vi "Create List Of FPGA in this Schedule.vi"(8 "error in (no error)":errorcluster, 11 "Schedule in":refnum<class "Schedule.lvclass">) -> (0 "error out":errorcluster, 3 "Schedule out":refnum<class "Schedule.lvclass">)   [LabVIEW 2020, in "TALOS.lvlib" / "Run Utilities.lvlib" / "Schedule.lvclass"]
doc: "Go over the entire schedule and create a list of Kaslis that are used in the Schedule"
uses:
  Schedule.lvclass
  Schedule.lvclass/Schedule.ctl
  Get List Of Kaslis in this Schedule.vi/21cbf78c-3c17-4340-8c34-790405437e2d.vi/d4db2432-cc9c-482c-8957-dac855435ef6.vi
  Get List Of Kaslis in this Schedule.vi/21cbf78c-3c17-4340-8c34-790405437e2d.vi/86fbf154-bd7b-49a2-8ab2-a837b2a95f24.vi
  Get List Of Kaslis in this Schedule.vi/21cbf78c-3c17-4340-8c34-790405437e2d.vi/3b95b01e-1ec2-4565-bcd9-7606a5281010.vi
  Get List Of Kaslis in this Schedule.vi/21cbf78c-3c17-4340-8c34-790405437e2d.vi/96a08935-737a-44b2-979c-a81d56408f7e.vi
  Get List Of Kaslis in this Schedule.vi/fc6b4163-bfed-4ba7-be7f-d257c96f9c4b.vi/c0db33a9-eb6c-44d9-b982-8563e05d2734.vi
  Get List Of Kaslis in this Schedule.vi/fc6b4163-bfed-4ba7-be7f-d257c96f9c4b.vi/ae3535a8-0066-4e8d-a5de-b07ac05a7c65.vi
  Get List Of Kaslis in this Schedule.vi/fc6b4163-bfed-4ba7-be7f-d257c96f9c4b.vi/dda8e586-731b-4197-ad83-6a4d05585a0a.vi
  Get List Of Kaslis in this Schedule.vi/21cbf78c-3c17-4340-8c34-790405437e2d.vi/d4db2432-cc9c-482c-8957-dac855435ef6.vi/6eaecd13-6e48-4772-a921-b51ebdf84d88.vi
  Get List Of Kaslis in this Schedule.vi/21cbf78c-3c17-4340-8c34-790405437e2d.vi/d4db2432-cc9c-482c-8957-dac855435ef6.vi/d2d5f2b7-06f4-47f6-971c-049c3fdbb653.vi
  Get List Of Kaslis in this Schedule.vi/21cbf78c-3c17-4340-8c34-790405437e2d.vi/3b95b01e-1ec2-4565-bcd9-7606a5281010.vi/6eaecd13-6e48-4772-a921-b51ebdf84d88.vi
  Get List Of Kaslis in this Schedule.vi/21cbf78c-3c17-4340-8c34-790405437e2d.vi/3b95b01e-1ec2-4565-bcd9-7606a5281010.vi/d2d5f2b7-06f4-47f6-971c-049c3fdbb653.vi
  Get List Of Kaslis in this Schedule.vi/21cbf78c-3c17-4340-8c34-790405437e2d.vi/96a08935-737a-44b2-979c-a81d56408f7e.vi/6eaecd13-6e48-4772-a921-b51ebdf84d88.vi
  Get List Of Kaslis in this Schedule.vi/21cbf78c-3c17-4340-8c34-790405437e2d.vi/96a08935-737a-44b2-979c-a81d56408f7e.vi/d2d5f2b7-06f4-47f6-971c-049c3fdbb653.vi
  Cell/Schedule Cell.lvclass
  <vilib>/Comparison/Less/Less Functor/Less Functor.lvclass
  b09dac26-fe60-4391-a7a8-81447650faa1.vi
  9bc96d9d-9184-4bd2-95c3-fe24546c86f6.vi
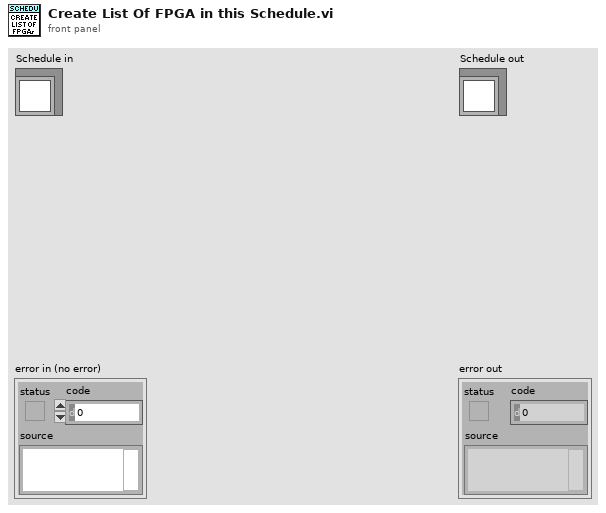
[diagram p1: front panel]
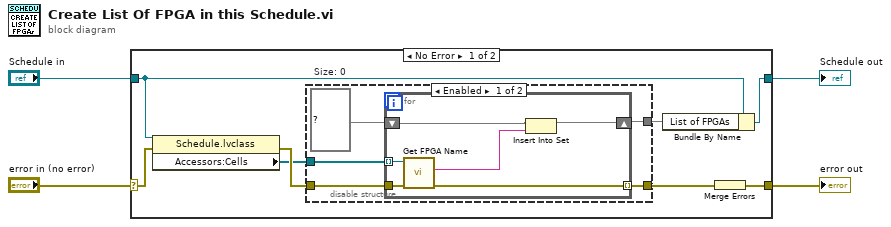
[diagram p0: block diagram]
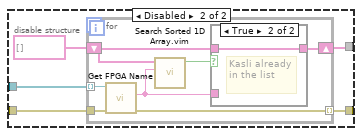
[diagram p2: hidden frame]
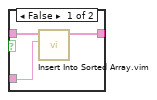
[diagram p3: hidden frame]
diagram:
  n1 = case shown="No Error" "error in (no error)" {
    selector: "error in (no error)" -> [w12 w41]
    tunnel: [w6 w41] -> w3
    tunnel: [w8 w40] -> w1
    tunnel: "Schedule in" -> [w9 w40]
    frame No Error {
      n2 = property class="Schedule.lvclass"(reference=w9, error in=w12) -> (error out=w11:errorcluster, "Accessors:Cells"=w10:refnum<class "Schedule Cell.lvclass">[])  [unwired: 1 out]
      n3 = disable-structure shown="Enabled" {
        disable-tunnel: w11 -> [w17 w28]
        disable-tunnel: w10 -> [w16 w27]
        disable-tunnel: [w15 w26] -> w7
        disable-tunnel: [w14 w24] -> w5
        frame Enabled {
          w13 = set{string} {}  # Size: 0
          n4 = for {
            tunnel: w16 -> [w22] mode=indexing
            tunnel: w17 -> [w23]
            shift-right: [w19] -> w14
            shift-left: w13 -> [w20]
            tunnel: [w21] -> w15 mode=indexing
            n5 = call-dynamic "Get FPGA Name.vi"("error in (no error)"=w23, "Schedule Cell in"=w22) -> ("error out"=w21:errorcluster, "FPGA Name"=w18:string)  [unwired: 7 in, 1 out]
            n6 = Insert Into Set(10:w18, 11:w20) -> (3:w19:set{string})  [unwired: 1 out]
          }
        }
        frame Disabled {
          n7 = for {
            tunnel: w27 -> [w34] mode=indexing
            tunnel: w28 -> [w35]
            shift-right: [w32] -> w24
            shift-left: string[] [] -> [w31]
            tunnel: [w33] -> w26 mode=indexing
            n8 = call-dynamic "Get FPGA Name.vi"("error in (no error)"=w35, "Schedule Cell in"=w34) -> ("error out"=w33:errorcluster, "FPGA Name"=w30:string)  [unwired: 7 in, 1 out]
            n9 = call "Search Sorted 1D Array.vim"("element"=w30, "sorted 1D array"=w31) -> ("found?"=w29:bool)  [unwired: 8 in, 1 out]
            n10 = case shown="True" w29 {
              tunnel: [w38 w39] -> w32
              tunnel: w31 -> [w37 w39]
              tunnel: w30 -> [w36 _]
              frame False {
                n11 = call "Insert Into Sorted Array.vim"("element"=w36, "sorted array in"=w37) -> ("sorted array out"=w38:string[])  [unwired: 9 in]
              }
              frame True {
                # "Kasli already in the list"
              }
            }
          }
        }
      }
      n12 = Bundle By Name(cluster=w9, "List of FPGAs"=w5) -> (w8:refnum<class "Schedule.lvclass">)
      n13 = Merge Errors(w7) -> (w6:errorcluster)
    }
    frame Error {
    }
  }
  "error out" <- w3
  "Schedule out" <- w1
